vi "串口通信1.vi"() -> ()   [LabVIEW 2018]
uses:
  <vilib>/Instr/_visa.llb/VISA Configure Serial Port (Instr).vi
panel:
  out "数字 3":dbl
  out "数字 2":dbl
  out "数字":dbl
  in  "baud rate (9600)":u32=9600
  out "读取缓冲区":string
  in  "VISA resource name":refnum<visa-resource-name> caption="VISA资源名称"
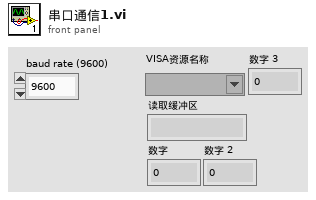
[diagram p1: front panel]
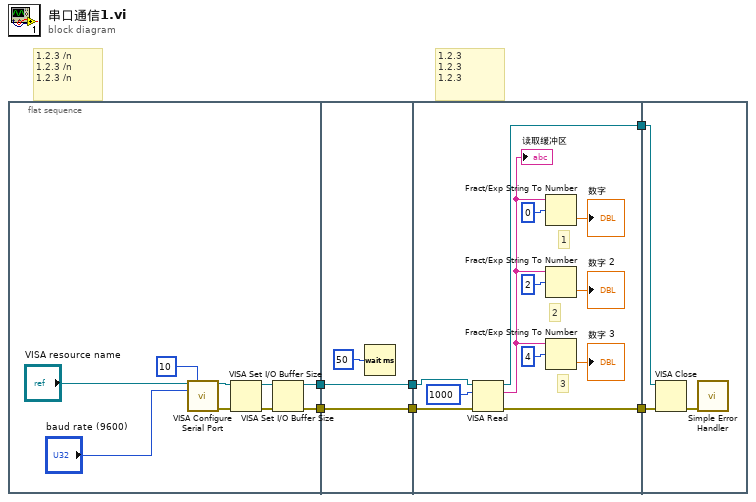
[diagram p0: block diagram]
diagram:
  # "1.2.3 \n1.2.3 \n1.2.3"
  # "1.2.3 /n\n1.2.3 /n\n1.2.3 /n"
  n1 = flat-sequence {
    tunnel: [w9] -> w5
    tunnel: [w8] -> w3
    tunnel: [w17] -> w6
    tunnel: w5 -> [w17]
    tunnel: [w16] -> w4
    tunnel: w3 -> [w16]
    tunnel: w6 -> [w30]
    tunnel: w4 -> [w29]
    tunnel: [w27] -> w2
    tunnel: [w26] -> w1
    tunnel: w2 -> [w33]
    tunnel: w1 -> [w32]
    frame #0 {
      n2 = call-poly "VISA Configure Serial Port"("VISA resource name"="VISA resource name", "timeout (10sec)"=u32 10, "baud rate (9600)"="baud rate (9600)") -> ("VISA resource name out"=w14:refnum<visa-resource-name>, "error out"=w12:errorcluster)  [unwired: 11 in]
      n3 = VISA Set I/O Buffer Size(VISA resource name=w14, error in (no error)=w12) -> (VISA resource name out=w13:refnum<visa-resource-name>, error out=w11:errorcluster)  [unwired: 2 in]
      n4 = VISA Set I/O Buffer Size(VISA resource name=w13, error in (no error)=w11) -> (VISA resource name out=w9:refnum<visa-resource-name>, error out=w8:errorcluster)  [unwired: 2 in]
    }
    frame #1 {
      n5 = Wait (ms)(milliseconds to wait=u32 50 ("等待时间（毫秒）")) -> ()  [unwired: 1 out]
    }
    frame #2 {
      # "3"
      # "2"
      # "1"
      n6 = VISA Read(VISA resource name=w30, byte count=u32 1000 ("字节总数"), error in (no error)=w29) -> (VISA resource name out=w27:refnum<visa-resource-name>, read buffer=w25:string, error out=w26:errorcluster)  [unwired: 1 out]
      "读取缓冲区" <- w25
      n7 = Fract/Exp String To Number(string=w25, offset=0 ("偏移量")) -> (number=→"数字":dbl)  [unwired: 2 in, 1 out]
      n8 = Fract/Exp String To Number(string=w25, offset=2 ("偏移量")) -> (number=→"数字 2":dbl)  [unwired: 2 in, 1 out]
      n9 = Fract/Exp String To Number(string=w25, offset=4 ("偏移量")) -> (number=→"数字 3":dbl)  [unwired: 2 in, 1 out]
    }
    frame #3 {
      n10 = VISA Close(VISA resource name=w33, error in (no error)=w32) -> (error out=w31:errorcluster)
      n11 = call <vilib>:"Simple Error Handler.vi"("error in (no error)"=w31) -> ()  [unwired: 4 in, 5 out]
    }
  }
